vi "transferVolume.vi"(5 "xyz order":bool, 7 "write to network stream":bool=TRUE, 8 "error in (no error)":errorcluster, 9 "num vol to sum":u32, 10 "network streaming queues":T2, 11 "Queues":T3) -> (0 "error out":errorcluster, 1 "volume update":bool, 2 "volumes sent":u32, 3 "last transfer timed out":bool, 4 "last volume sent":T1, 6 "n disp vol":i32)   [LabVIEW 2010]
uses:
  internal_queues.ctl
  line_info.ctl
  volume_with_lines.ctl
  volume_info.ctl
  kalman_result_scaled.ctl
  location3D.ctl
  spot location.ctl
  network_streaming_queues_cluster.ctl
  scan_specification_cluster.ctl
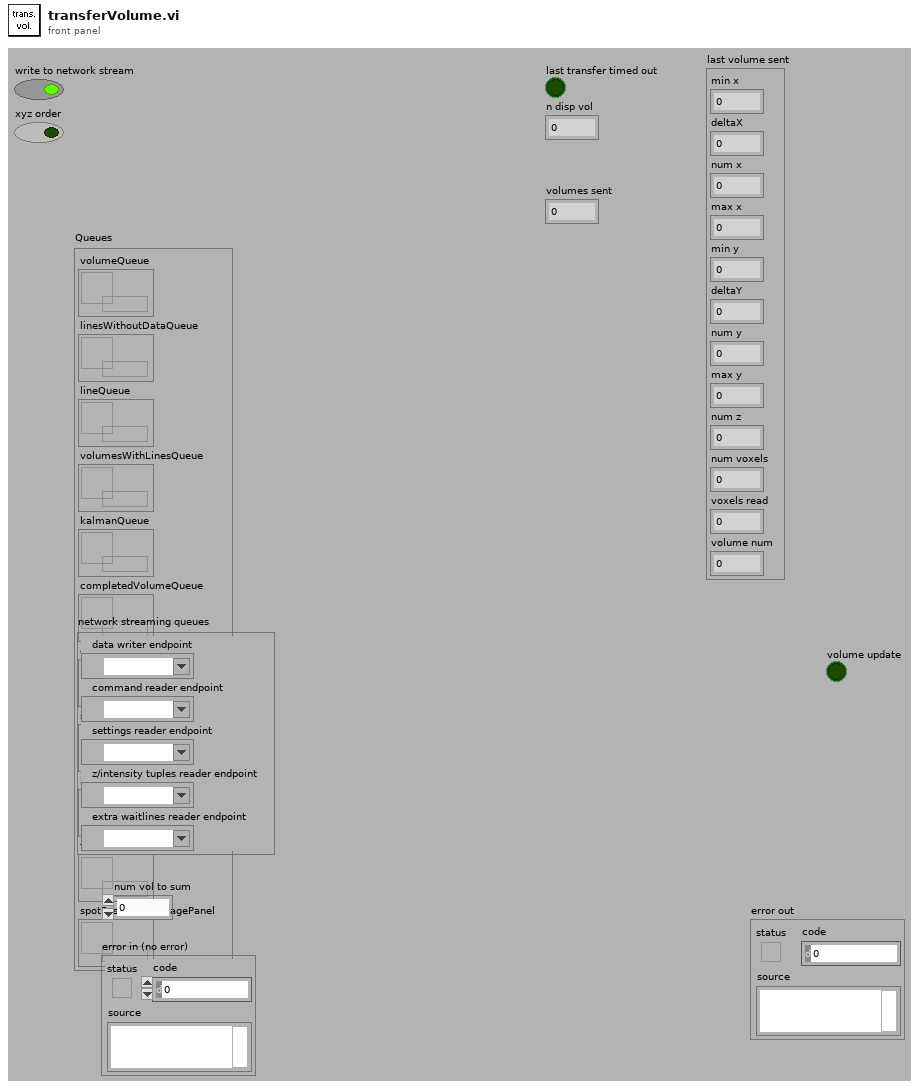
[diagram p1: front panel]
types:
  T1 = cluster{"min x":i16, "deltaX":dbl, "num x":u32, "max x":i16, "min y":i16, "deltaY":dbl, "num y":u32, "max y":i16, "num z":u32, "num voxels":u32, "voxels read":u32, "volume num":u32}
  T2 = typedef "network_streaming_queues_cluster.ctl" = cluster{"data writer endpoint":refnum<k21>, "command reader endpoint":refnum<k21>, "settings reader endpoint":refnum<k21>, "z/intensity tuples reader endpoint":refnum<k21>, "extra waitlines reader endpoint":refnum<k21>}
  T3 = typedef "internal_queues.ctl" = cluster{"volumeQueue":refnum<queue>, "linesWithoutDataQueue":refnum<queue>, "lineQueue":refnum<queue>, "volumesWithLinesQueue":refnum<queue>, "kalmanQueue":refnum<queue>, "completedVolumeQueue":refnum<queue>, "displayVolumeQueue":refnum<queue>, "scanLocationsQueue":refnum<queue>, "kalmanToDisplayPanel":refnum<queue>, "focalPositionQueue":refnum<queue>, "spotPositionsToImagePanel":refnum<queue>}
  T4 = cluster{"volume info":cluster{"min x":i16, "deltaX":dbl, "num x":u32, "max x":i16, "min y":i16, "deltaY":dbl, "num y":u32, "max y":i16, "num z":u32, "num voxels":u32, "voxels read":u32, "volume num":u32}, "buffer":u32[]}
  T5 = cluster{"Numeric":u32, "Numeric":u32, "Numeric":u32, "Numeric":u32}
  T6 = cluster{"image":u32[][][], "image":u32[][][], u32[][][], u32[][][]}
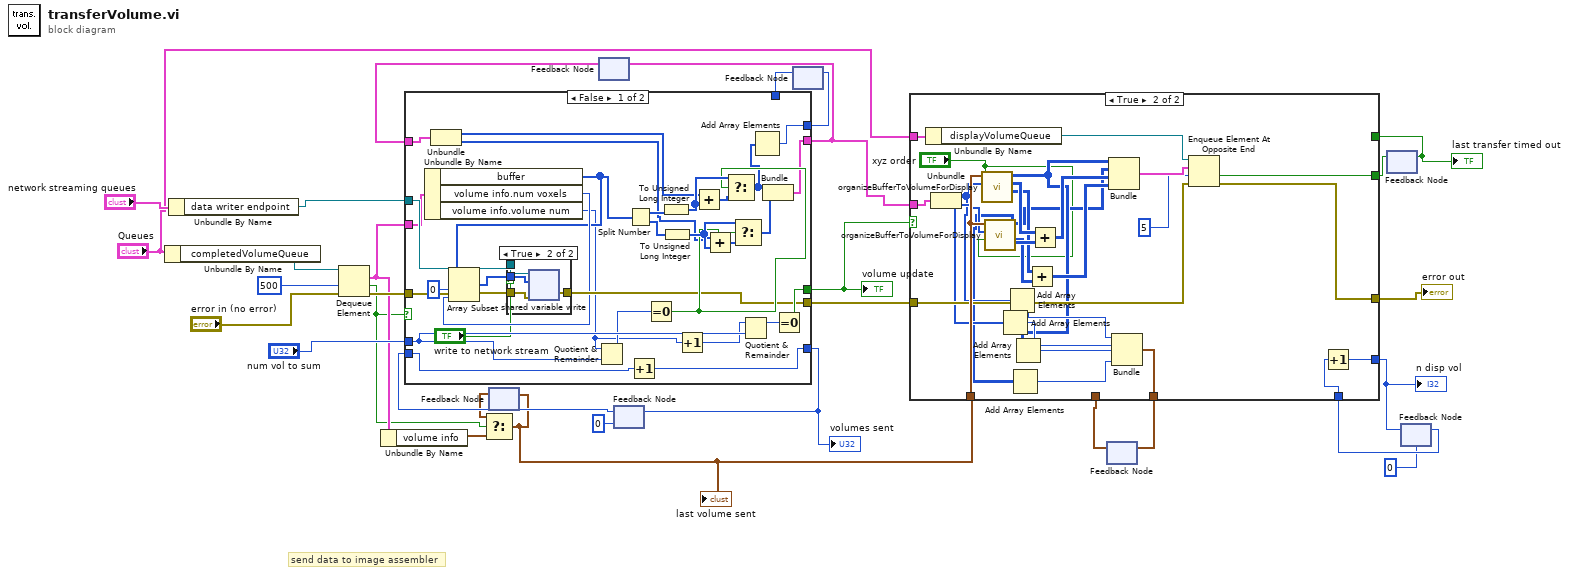
[diagram p0: block diagram]
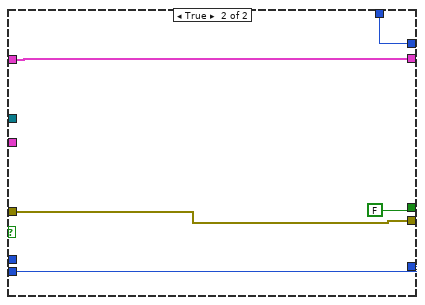
[diagram p4: hidden frame]
diagram:
  # "send data to image assembler"
  n1 = Unbundle By Name("Queues") -> ("completedVolumeQueue"=w30:refnum<queue>)
  n2 = Unbundle By Name("network streaming queues") -> ("data writer endpoint"=w26:refnum<k21>)
  n3 = Dequeue Element(queue=w30, timeout in ms (-1)=500, error in (no error)="error in (no error)") -> (element=w19:T4, timed out?=w17:bool, error out=w25:errorcluster)  [unwired: 1 out]
  n4 = Unbundle By Name(w19) -> ("volume info"=w18:T1)
  n5 = feedback #1() -> (w16:T1)  [unwired: 1 in]
  n6 = Select(t=w16, s=w17, f=w18) -> (s? t:f=w15:T1)
  "last volume sent" <- w15
  n7 = feedback-in #1(w15) -> ()
  n8 = feedback #2() -> (w20:cluster{u32[], u32[]})  [unwired: 1 in]
  n9 = feedback #3(u32 0) -> (w22:u32)
  n10 = feedback #4() -> (w1:u32)  [unwired: 1 in]
  n11 = case shown="False" w17 {
    tunnel: w19 -> [w59 _]
    tunnel: w26 -> [w61 _]
    tunnel: w25 -> [w60 w68]
    tunnel: "num vol to sum" -> [w45 _]
    tunnel: [w46 w69] -> w23
    tunnel: w22 -> [w37 w69]
    tunnel: [w50 w71] -> w10
    tunnel: w20 -> [w49 w71]
    tunnel: [w43 FALSE] -> w14
    tunnel: [w42 w68] -> w13
    tunnel: [w32 w67] -> w2
    tunnel: w1 -> [_ w67]
    frame False {
      n12 = Unbundle By Name(w59) -> ("buffer"=w38:u32[], "volume info.num voxels"=w39:u32, "volume info.volume num"=w35:u32)
      n13 = Unbundle(w49) -> (w48:u32[], w47:u32[])
      n14 = Array Subset(array=w38, index=0, length=w39) -> (w41:u32[])
      n15 = case shown="True" "write to network stream" {
        tunnel: w61 -> [_ w66]
        tunnel: w60 -> [w62 w65]
        tunnel: [w62 w64] -> w42
        tunnel: w41 -> [_ w63]
        frame False {
        }
        frame True {
          n16 = shared-variable-write(w66, w65, w63) -> (w64:errorcluster)  [unwired: 1 in, 2 out]
        }
      }
      n17 = Quotient & Remainder(x=w35, y=w45) -> (x-y*floor(x/y)=w36:u32)  [unwired: 1 out]
      n18 = Split Number(x=w38) -> (hi(x)=w58:u16[], lo(x)=w57:u16[])
      n19 = Increment(x=w37) -> (x+1=w46:u32)
      n20 = Equal To 0?(x=w36) -> (x = 0?=w52:bool)
      n21 = To Unsigned Long Integer(number=w58) -> (unsigned 32bit integer=w55:u32[])
      n22 = To Unsigned Long Integer(number=w57) -> (unsigned 32bit integer=w53:u32[])
      n23 = Increment(x=w35) -> (x+1=w34:u32)
      n24 = Add(x=w48, y=w55) -> (x+y=w56:u32[])
      n25 = Add(x=w47, y=w53) -> (x+y=w54:u32[])
      n26 = Select(t=w55, s=w52, f=w56) -> (s? t:f=w33:u32[])
      n27 = Select(t=w53, s=w52, f=w54) -> (s? t:f=w51:u32[])
      n28 = Quotient & Remainder(x=w34, y=w45) -> (x-y*floor(x/y)=w44:u32)  [unwired: 1 out]
      n29 = Add Array Elements(numeric array=w33) -> (sum=w32:u32)
      n30 = Bundle(w33, w51) -> (w50:cluster{u32[], u32[]})  [unwired: 1 in]
      n31 = Equal To 0?(x=w44) -> (x = 0?=w43:bool)
    }
    frame True {
    }
  }
  "volume update" <- w14
  "volumes sent" <- w23
  n32 = feedback-in #2(w10) -> ()
  n33 = feedback-in #3(w23) -> ()
  n34 = feedback-in #4(w2) -> ()
  n35 = feedback #5() -> (w8:T5)  [unwired: 1 in]
  n36 = feedback #6() -> (w6:bool)  [unwired: 1 in]
  "last transfer timed out" <- w6
  n37 = feedback #7(0) -> (w4:i32)
  n38 = case shown="True" w14 {
    tunnel: w15 -> [_ w102]
    tunnel: w10 -> [_ w95]
    tunnel: w13 -> [w75 w91]
    tunnel: "Queues" -> [_ w94]
    tunnel: [w75 w90] -> w11
    tunnel: [w74 w80] -> w9
    tunnel: w8 -> [w74 _]
    tunnel: [w73 w79] -> w7
    tunnel: w6 -> [w73 _]
    tunnel: [w72 w78] -> w5
    tunnel: w4 -> [w72 w77]
    frame False {
    }
    frame True {
      n39 = Unbundle By Name(w94) -> ("displayVolumeQueue"=w92:refnum<queue>)
      n40 = Unbundle(w95) -> (w87:u32[], w88:u32[])
      n41 = call "organizeBufferToVolumeForDisplay.vi"("xyz mode"="xyz order", "buffer"=w87, "volume info"=w102) -> ("fb only (image if no ff/fb)"=w98:u32[][][], "ff only (0 if no ff/fb)"=w101:u32[][][], "image"=w84:u32[][][])  [unwired: 6 in]
      n42 = call "organizeBufferToVolumeForDisplay.vi"("xyz mode"="xyz order", "buffer"=w88, "volume info"=w102) -> ("fb only (image if no ff/fb)"=w99:u32[][][], "ff only (0 if no ff/fb)"=w100:u32[][][], "image"=w82:u32[][][])  [unwired: 6 in]
      n43 = Add Array Elements(numeric array=w88) -> (sum=w85:u32)
      n44 = Add Array Elements(numeric array=w87) -> (sum=w86:u32)
      n45 = Add Array Elements(numeric array=w82) -> (sum=w81:u32)
      n46 = Add Array Elements(numeric array=w84) -> (sum=w83:u32)
      n47 = Add(x=w98, y=w99) -> (x+y=w96:u32[][][])
      n48 = Add(x=w101, y=w100) -> (x+y=w97:u32[][][])
      n49 = Bundle("image"=w84, "image"=w82, w97, w96) -> (w93:T6)  [unwired: 1 in]
      n50 = Bundle("Numeric"=w86, "Numeric"=w85, "Numeric"=w83, "Numeric"=w81) -> (w80:T5)  [unwired: 1 in]
      n51 = Enqueue Element At Opposite End(queue=w92, element=w93, timeout in ms (-1)=5, error in (no error)=w91) -> (timed out?=w79:bool, error out=w90:errorcluster)  [unwired: 1 out]
      n52 = Increment(x=w77) -> (x+1=w78:i32)
    }
  }
  "error out" <- w11
  "n disp vol" <- w5
  n53 = feedback-in #5(w9) -> ()
  n54 = feedback-in #6(w7) -> ()
  n55 = feedback-in #7(w5) -> ()
